vi "DC Parameter.vi"(8 "error in (no error)":errorcluster, 11 "BK-Precision in":refnum<class "BK-Precision.lvclass">) -> (0 "error out":errorcluster, 2 "DC Parameter":dbl[](array[numeric]), 3 "BK-Precision out":refnum<class "BK-Precision.lvclass">)   [LabVIEW 2016, in "DC PWS.lvlib" / "BK-Precision.lvclass"]
uses:
  BK-Precision.lvclass
  BK-Precision.lvclass/BK-Precision.ctl
  <instrlib>/BK Precision 911X Series/BK Precision 911X Series.lvlib
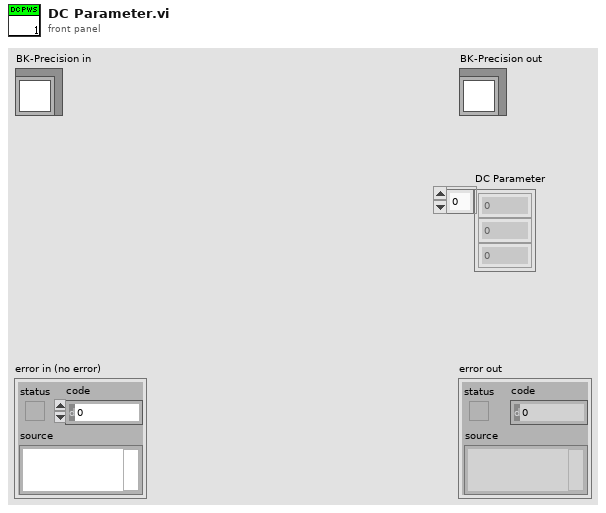
[diagram p1: front panel]
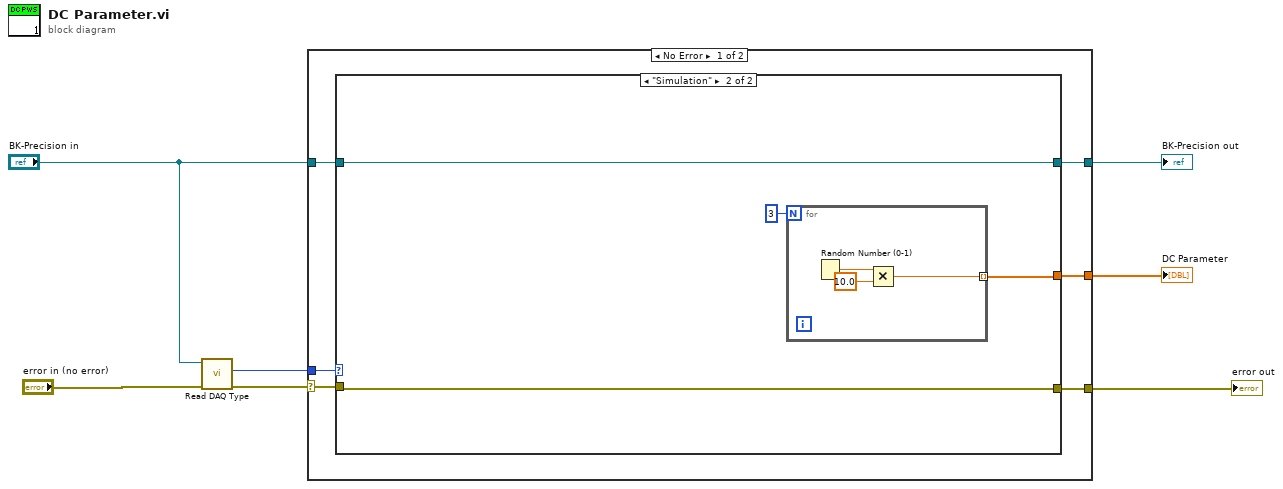
[diagram p0: block diagram]
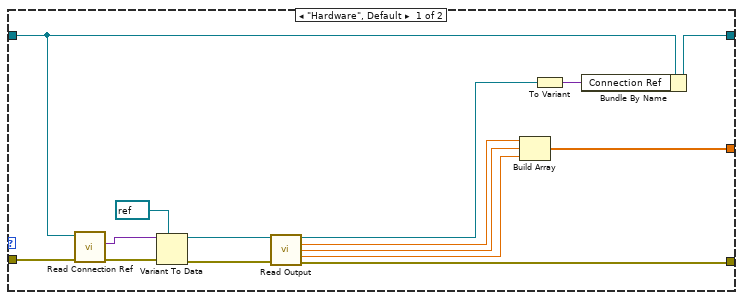
[diagram p2: hidden frame]
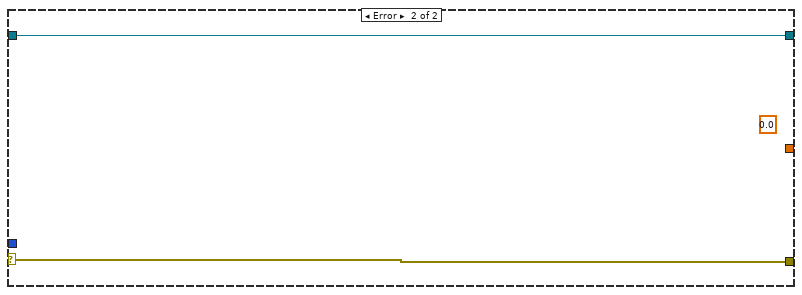
[diagram p3: hidden frame]
diagram:
  n1 = call "Read DAQ Type.vi"("error in (no error)"="error in (no error)", "BK-Precision in"="BK-Precision in") -> ("error out"=w7:errorcluster, "Type"=w6:enum16{"Hardware", "Simulation"})  [unwired: 7 in, 1 out]
  n2 = case shown="No Error" w7 {
    selector: w7 -> [w11 w36]
    tunnel: w6 -> [w13 _]
    tunnel: "BK-Precision in" -> [w12 w37]
    tunnel: [w10 w37] -> w2
    tunnel: [w9 w36] -> w5
    tunnel: [w8 _] -> w1
    frame No Error {
      n3 = case shown="\"Simulation\"" w13 {
        tunnel: w12 -> [w27 w32]
        tunnel: w11 -> [w28 w31]
        tunnel: [w21 w32] -> w10
        tunnel: [w19 w31] -> w9
        tunnel: [w15 w29] -> w8
        frame "Hardware", Default {
          n4 = call "Read Connection Ref.vi"("error in (no error)"=w28, "BK-Precision in"=w27) -> ("error out"=w26:errorcluster, "Conn Ref"=w25:variant)  [unwired: 7 in, 1 out]
          n5 = Variant To Data(error in=w26, type=refnum<visa-resource-name> refnum ("VISA resource name"), Variant=w25) -> (data=w23:refnum<visa-resource-name>, error out=w22:errorcluster)
          n6 = call <instrlib>:"Read Output.vi"("VISA resource name"=w23, "error in (no error)"=w22) -> ("VISA resource name out"=w20:refnum<visa-resource-name>, "Actual Voltage Level (V)"=w18:dbl, "Actual Current Level (A)"=w17:dbl, "Actual Power Level (W)"=w16:dbl, "error out"=w19:errorcluster)  [unwired: 9 in]
          n7 = Build Array(w18, w17, w16) -> (w15:dbl[])
          n8 = To Variant(anything=w20) -> (Variant=w14:variant)
          n9 = Bundle By Name(cluster=w27, "Connection Ref"=w14) -> (w21:refnum<class "BK-Precision.lvclass">)
        }
        frame "Simulation" {
          n10 = for {
            N: 3 -> [_]
            tunnel: [w33] -> w29 mode=indexing
            n11 = Random Number (0-1)() -> (number: 0 to 1=w35:dbl)
            n12 = Multiply(x=w35, y=10.0) -> (x*y=w33:dbl)
          }
        }
      }
    }
    frame Error {
      (unwired) 0.0 ("Actual Power Level (W)")
    }
  }
  "error out" <- w5
  "BK-Precision out" <- w2
  "DC Parameter" <- w1
